vi "convert_string_to_boolean.vi"(4 "String in":string) -> (1 "boolean value out":bool)   [LabVIEW 2022 SP3, in "hmp4000_rsidr_core.lvlib"]
uses:
  hmp4000_rsidr_core.lvlib
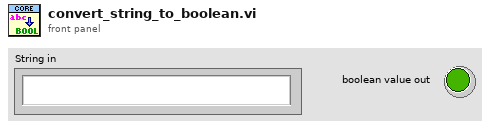
[diagram p1: front panel]
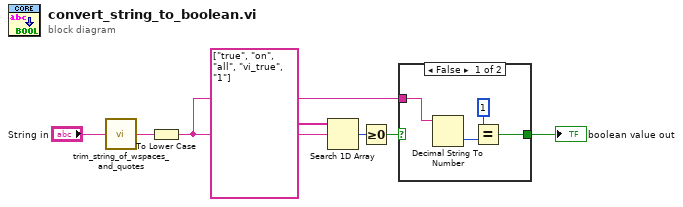
[diagram p0: block diagram]
diagram:
  n1 = call "trim_string_of_wspaces_and_quotes.vi"("String in"="String in") -> ("String out"=w1:string)  [unwired: 4 in]
  n2 = To Lower Case(string=w1) -> (all lower case string=w3:string)
  n3 = Search 1D Array(1D array=string[] ["true", "on", "all", "vi_true", "1"], element=w3) -> (index of element=w6:i32)  [unwired: 1 in]
  n4 = Greater Or Equal To 0?(x=w6) -> (x >= 0?=w5:bool)
  n5 = case shown="False" w5 {
    selector: w5 -> [_ w12]
    tunnel: [w8 w12] -> w4
    tunnel: w3 -> [w9 _]
    frame False {
      n6 = Decimal String To Number(string=w9) -> (number=w11:i32)  [unwired: 2 in, 1 out]
      n7 = Equal?(x=1, y=w11) -> (x = y?=w8:bool)
    }
    frame True {
    }
  }
  "boolean value out" <- w4
